vi "Pupil_Parameters.vi"(4 "img_cols":u16, 6 "img_rows":u16, 8 "8-bit pixmap":u8[][](array[numeric]), 9 "N_pts":u8, 10 "GB":u8, 11 "AT":u8) -> (0 "Radius_STD":i16, 1 "Radius":i16, 2 "Pup_y":i16, 3 "Pup_x":i16)   [LabVIEW 2018]
uses:
  Program_v2.3/dll/Pupil_cpp_dll_for_LV.dll
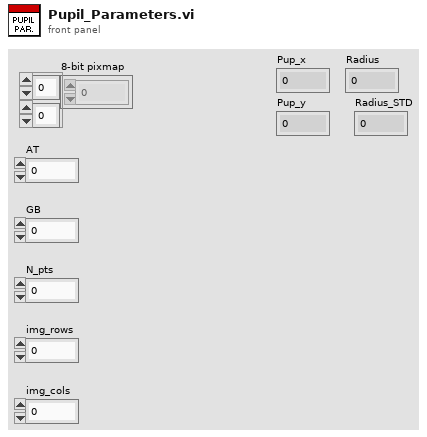
[diagram p1: front panel]
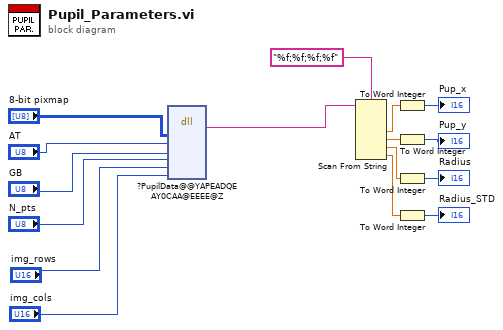
[diagram p0: block diagram]
diagram:
  n1 = dll-call lib="D:/Program_v2.3/dll/Pupil_cpp_dll_for_LV.dll" fn="?PupilData@@YAPEADQEAY0CAA@EEEE@Z"("arr"="8-bit pixmap", "AT"="AT", "GB"="GB", "N_ps"="N_pts", "img_rows"="img_rows", "img_cols"="img_cols") -> (error out=w4:errorcluster, "C_pupil_data"=w8:string)  [unwired: 9 in, 1 out]
  n2 = Scan From String(format string="%f;%f;%f;%f", input string=w8) -> (output 1=w16:dbl, output 2=w15:dbl, output 3=w14:dbl, output 4=w13:dbl)  [unwired: 6 in, 3 out]
  n3 = To Word Integer(number=w16) -> (16bit integer=→"Pup_x":i16)
  n4 = To Word Integer(number=w15) -> (16bit integer=→"Pup_y":i16)
  n5 = To Word Integer(number=w14) -> (16bit integer=→"Radius":i16)
  n6 = To Word Integer(number=w13) -> (16bit integer=→"Radius_STD":i16)
